vi "GetSweepConfigurationByChannel.vi"(10 "AssetNodes":T1[](array[typedef]), 11 "AssetNodeId":string) -> (2 "total number of points":i32, 3 "sweep freq list":cluster{"frequency":dbl, "bandwidth":dbl}[](array[cluster]))   [LabVIEW 2017, in "EmsaAcquisition.lvlib"]
uses:
  <vilib>/addons/InsightCM/Devices/Shared/Emsa/EmsaAcquisition/EmsaAcquisition.lvlib
  <vilib>/addons/InsightCM/MessageBus/Base/controls/AssetNode.ctl
  <vilib>/addons/InsightCM/MessageBus/Base/controls/AssetState.ctl
  <vilib>/addons/InsightCM/MessageBus/Base/controls/KeyValuePair.ctl
  <vilib>/addons/InsightCM/MessageBus/Base/controls/OperatingState.ctl
  <vilib>/addons/InsightCM/MessageBus/Base/controls/Trigger.ctl
  <vilib>/addons/InsightCM/MessageBus/Base/controls/Condition.ctl
  <vilib>/addons/InsightCM/MessageBus/Base/controls/Metric.ctl
  <vilib>/addons/InsightCM/MessageBus/Base/controls/TrendAlarmRule.ctl
  <vilib>/addons/InsightCM/MessageBus/Base/controls/TrendAlarmLevel.ctl
  <vilib>/addons/InsightCM/MessageBus/Base/controls/AlarmAction.ctl
  <vilib>/addons/InsightCM/MessageBus/Base/controls/AssetNodeReference.ctl
  <vilib>/addons/InsightCM/Utilities/PropertyHelpers/PropertyHelpers.lvlib
  <vilib>/addons/InsightCM/Utilities/DeviceModelHelpers/DeviceModelHelpers.lvlib
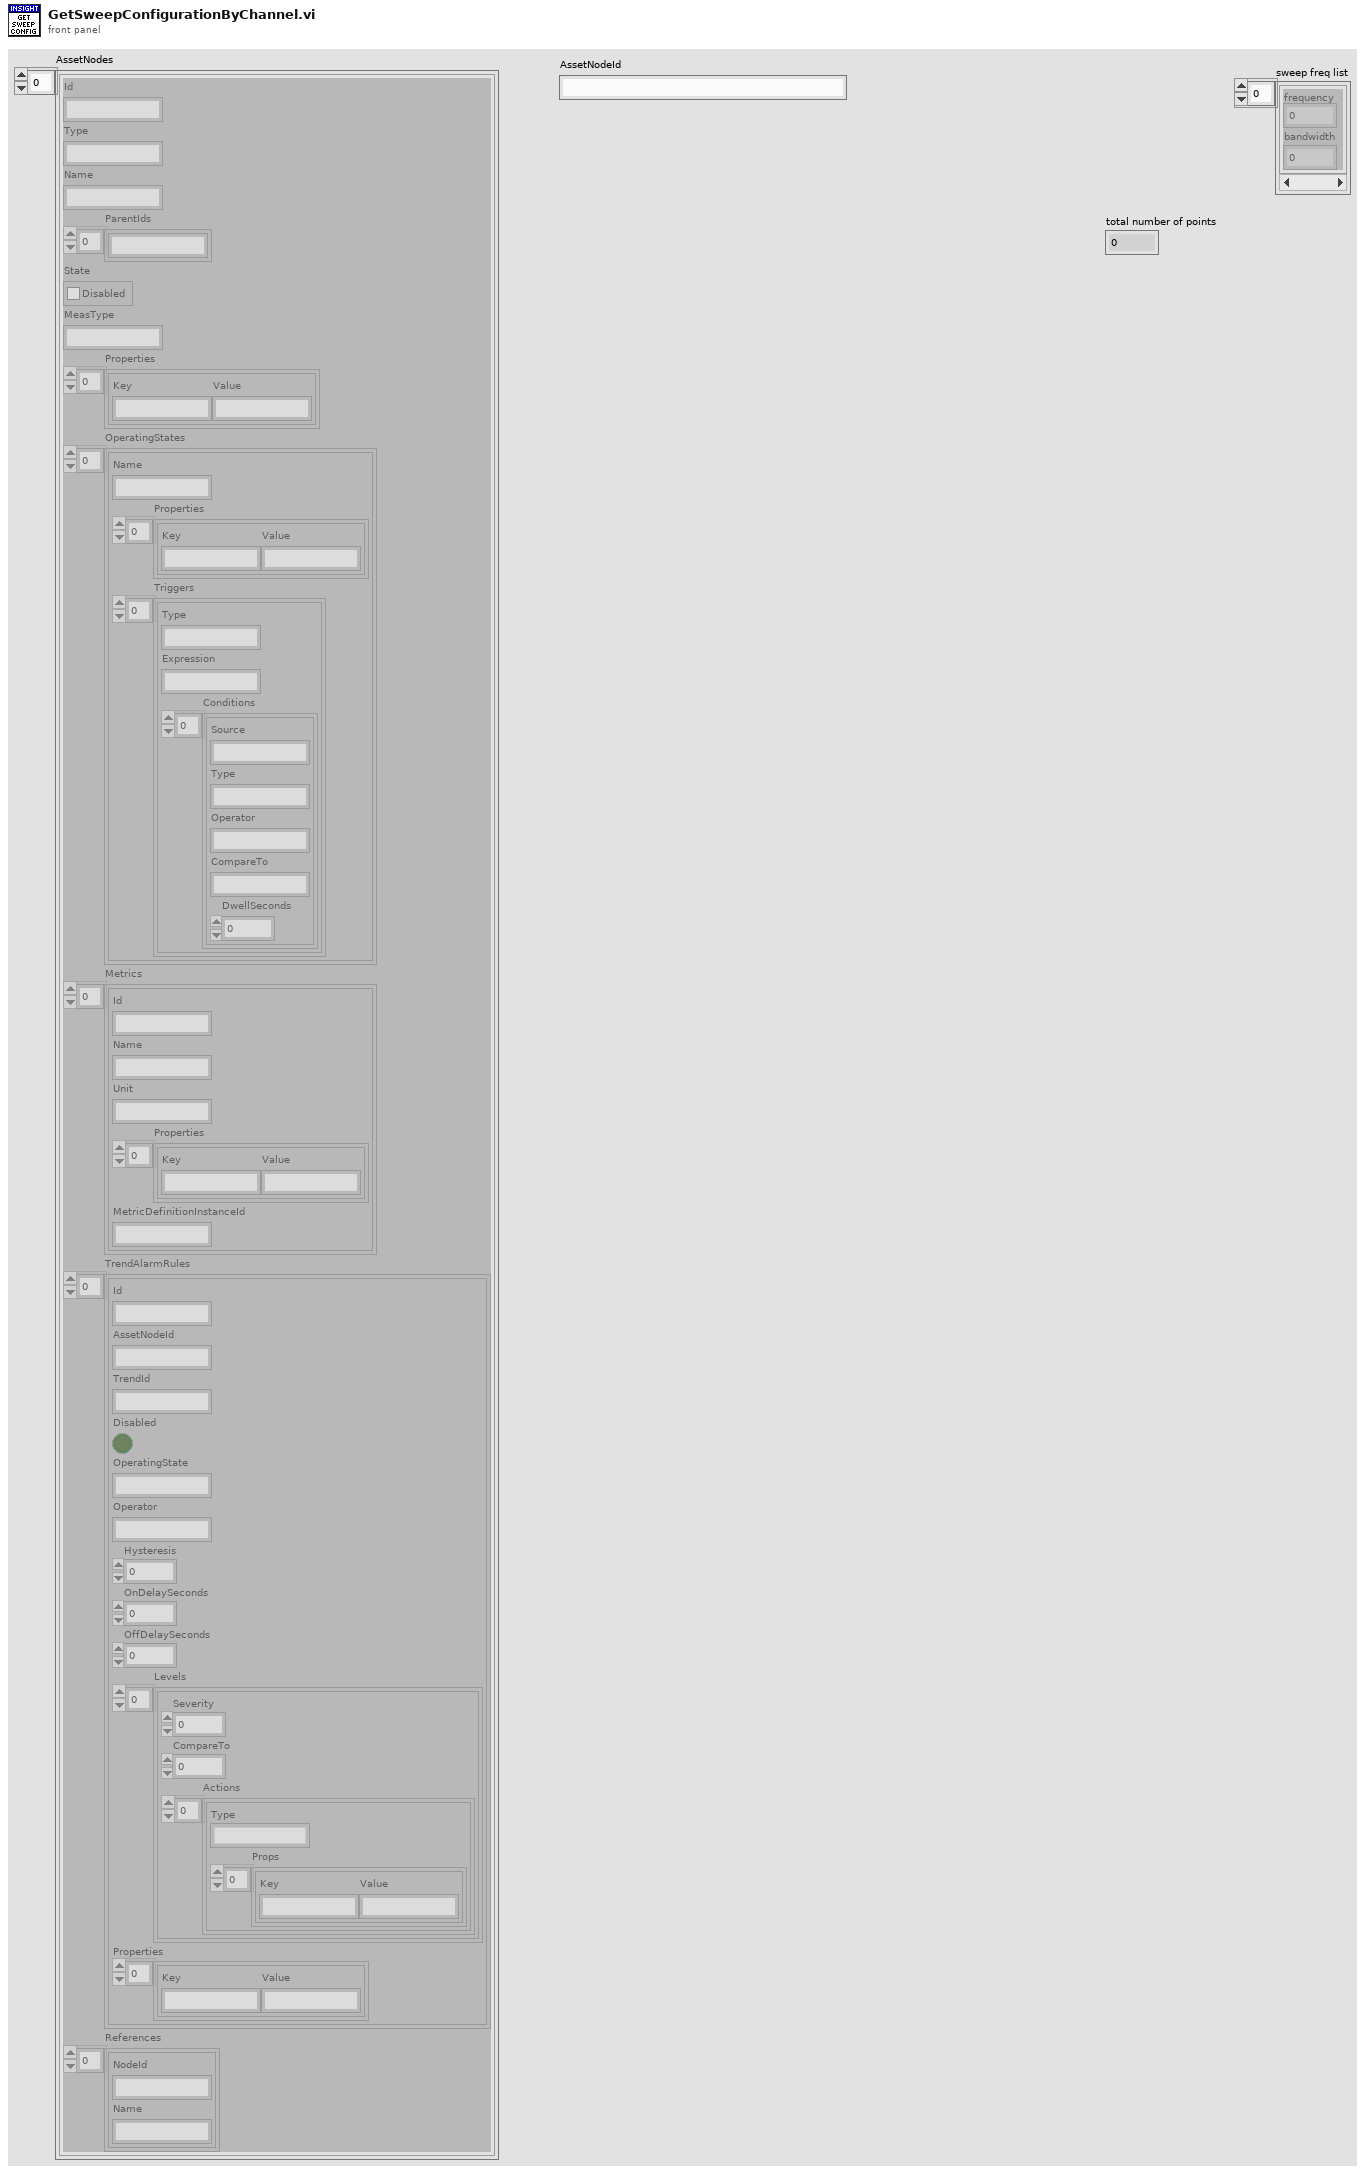
[diagram p1: front panel]
types:
  T1 = typedef "AssetNode.ctl" = cluster{"Id":string, "Type":string, "Name":string, "ParentIds":string[], "State":T2, "MeasType":string, "Properties":T3[], "OperatingStates":T4[], "Metrics":T7[], "TrendAlarmRules":T8[], "References":T11[]}
  T2 = typedef "AssetState.ctl" = cluster{"Disabled":bool}
  T3 = typedef "KeyValuePair.ctl" = cluster{"Key":string, "Value":string}
  T4 = typedef "OperatingState.ctl" = cluster{"Name":string, "Properties":T3[], "Triggers":T5[]}
  T5 = typedef "Trigger.ctl" = cluster{"Type":string, "Expression":string, "Conditions":T6[]}
  T6 = typedef "Condition.ctl" = cluster{"Source":string, "Type":string, "Operator":string, "CompareTo":string, "DwellSeconds":dbl}
  T7 = typedef "Metric.ctl" = cluster{"Id":string, "Name":string, "Unit":string, "Properties":T3[], "MetricDefinitionInstanceId":string}
  T8 = typedef "TrendAlarmRule.ctl" = cluster{"Id":string, "AssetNodeId":string, "TrendId":string, "Disabled":bool, "OperatingState":string, "Operator":string, "Hysteresis":dbl, "OnDelaySeconds":dbl, "OffDelaySeconds":dbl, "Levels":T9[], "Properties":T3[]}
  T9 = typedef "TrendAlarmLevel.ctl" = cluster{"Severity":i32, "CompareTo":dbl, "Actions":T10[]}
  T10 = typedef "AlarmAction.ctl" = cluster{"Type":string, "Props":T3[]}
  T11 = typedef "AssetNodeReference.ctl" = cluster{"NodeId":string, "Name":string}
  T12 = cluster{"num points":i32, "start freq":dbl, "stop freq":dbl, "bandwidth":dbl}
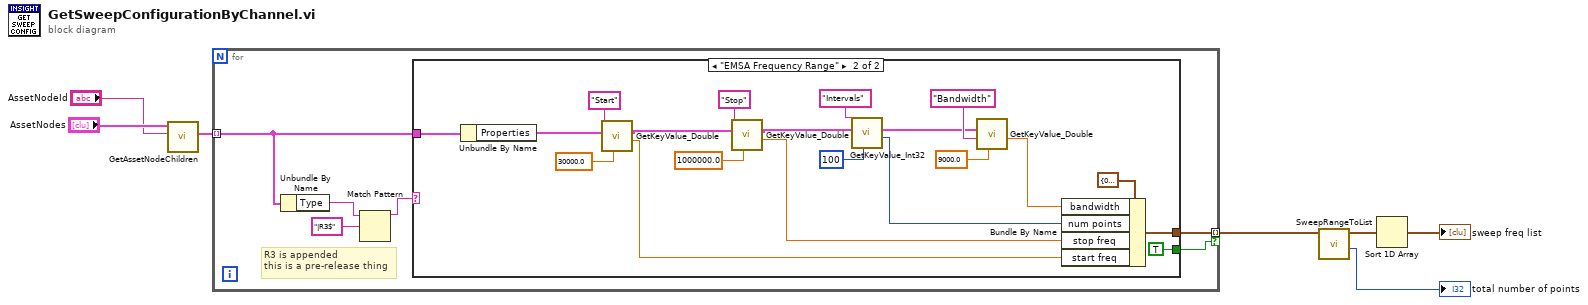
[diagram p0: block diagram]
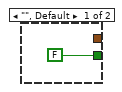
[diagram p2: hidden frame]
diagram:
  n1 = call <vilib>:"GetAssetNodeChildren.vi"("node id"="AssetNodeId", "nodes in"="AssetNodes") -> ("Children"=w2:T1[])  [unwired: 8 in, 1 out]
  n2 = for {
    tunnel: [w13] -> w7 mode=indexing if=w8
    tunnel: w2 -> [w12] mode=indexing
    # "R3 is appended\nthis is a pre-release thing"
    n3 = Unbundle By Name(w12) -> ("Type"=w10:string)
    n4 = Match Pattern(string=w10, regular expression="|R3$") -> (before substring=w9:string)  [unwired: 1 in, 3 out]
    n5 = case shown="\"EMSA Frequency Range\"" w9 {
      tunnel: [_ w18] -> w13
      tunnel: w12 -> [_ w17]
      tunnel: [FALSE TRUE] -> w8
      frame "", Default {
      }
      frame "EMSA Frequency Range" {
        n6 = Unbundle By Name(w17) -> ("Properties"=w16:T3[])
        n7 = call <vilib>:"GetKeyValue_Double.vi"("default"=30000.0, "key"="Start", "key value pairs"=w16) -> ("value"=w19:dbl, "key value pairs out"=w30:T3[])  [unwired: 6 in, 1 out]
        n8 = call <vilib>:"GetKeyValue_Double.vi"("default"=1000000.0, "key"="Stop", "key value pairs"=w30) -> ("value"=w20:dbl, "key value pairs out"=w25:T3[])  [unwired: 6 in, 1 out]
        n9 = call <vilib>:"GetKeyValue_Int32.vi"("default"=100, "key"="Intervals", "key value pairs"=w25) -> ("value"=w21:i32, "key value pairs out"=w26:T3[])  [unwired: 6 in, 1 out]
        n10 = call <vilib>:"GetKeyValue_Double.vi"("default"=9000.0, "key"="Bandwidth", "key value pairs"=w26) -> ("value"=w22:dbl)  [unwired: 6 in, 2 out]
        n11 = Bundle By Name(cluster=T12 {"num points"=0, "start freq"=0.0, "stop freq"=0.0, "bandwidth"=0.0} ("frequency sweep"), "bandwidth"=w22, "num points"=w21, "stop freq"=w20, "start freq"=w19) -> (w18:T12)
      }
    }
  }
  n12 = call <vilib>:"SweepRangeToList.vi"("sweep ranges"=w7) -> ("totalNumberOfPoints"=→"total number of points":i32, "sweep freq list"=w6:cluster{"frequency":dbl, "bandwidth":dbl}[])  [unwired: 9 in]
  n13 = Sort 1D Array(array=w6) -> (sorted array=→"sweep freq list":cluster{"frequency":dbl, "bandwidth":dbl}[])
